vi "Extra_Motor.vi"(7 "refnum name":string="My Motor RefNum", 8 "Back Speed":dbl, 9 "For Speed":dbl, 10 "Backward":bool, 11 "Forward":bool) -> ()   [LabVIEW 2017]
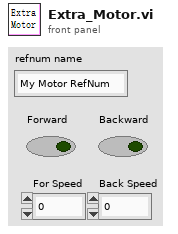
[diagram p1: front panel]
types:
  T1 = typedef "WPI_MotorControlDeviceRef.ctl" = cluster{"DeviceStatus":errorcluster, "Type":T2, "PWM":cluster{"PWM Channel":T3, "DeadBand":T4}, "CAN":cluster{"Device Number":u8, "SetOutput VI Ref":variant, "GetOutput VI Ref":variant, "Enable VI Ref":variant, "Disable VI Ref":variant, "Data":variant}, "Invert":bool, "DIO PWM":cluster{"PWM \"Enable\" Channel":T3, "DIOChannel":T5, "PWM Rate":dbl}}
  T2 = typedef "WPI_MotorControlType.ctl" = enum16{"PWM", "CAN", "DIO PWM"}
  T3 = typedef "FPGA_DIOPWMChannel.ctl" = enum8{"PWM 0", "PWM 1", "PWM 2", "PWM 3", "PWM 4", "PWM 5", "PWM 6", "PWM 7", "PWM 8", "PWM 9", "PWM MXP 0", "PWM MXP 1", "PWM MXP 2", "PWM MXP 3", "PWM MXP 4", "PWM MXP 5", "PWM MXP 6", "PWM MXP 7", "PWM MXP 8", "PWM MXP 9", "Invalid"}
  T4 = typedef "WPI_PWMDeadband.ctl" = cluster{"Name":string, "maxPositivePwm":i32, "minPositivePwm":i32, "centerPwm":i32, "maxNegativePwm":i32, "minNegativePwm":i32, "angularRange":u16}
  T5 = typedef "FPGA_DIOChannel.ctl" = enum8{"DIO 0", "DIO 1", "DIO 2", "DIO 3", "DIO 4", "DIO 5", "DIO 6", "DIO 7", "DIO 8", "DIO 9", "DIO MXP 0", "DIO MXP 1", "DIO MXP 2", "DIO MXP 3", "DIO MXP 4", "DIO MXP 5", "DIO MXP 6", "DIO MXP 7", "DIO MXP 8", "DIO MXP 9", "DIO MXP 10", "DIO MXP 11", "DIO MXP 12", "DIO MXP 13", "DIO MXP 14", "DIO MXP 15", "SPI Port CS1", "SPI Port CS2", "SPI Port CS3", "SPI Port MISO", "SPI Port MOSI", "Invalid"}
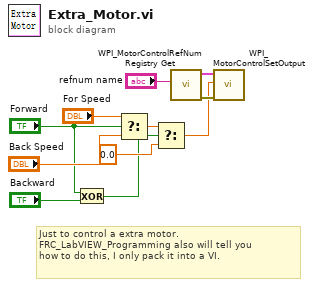
[diagram p0: block diagram]
diagram:
  # "Just to control a extra motor.\nFRC_LabVIEW_Programming also will tell you\nhow to do this, I only pack it into a VI."
  n1 = Exclusive Or(1:"Backward", 2:"Forward") -> (0:w4:bool)
  n2 = Select(t="For Speed", s="Forward", f="Back Speed") -> (s? t:f=w8:dbl)
  n3 = Select(t=w8, s=w4, f=0.0) -> (s? t:f=w1:dbl)
  n4 = call <vilib>:"WPI_MotorControlRefNum Registry Get.vi"("refnum name"="refnum name") -> ("error out"=w3:errorcluster, "MotorControlDevRef"=w2:T1)  [unwired: 9 in]
  n5 = call <vilib>:"WPI_MotorControlSetOutput.vi"("error in (no error)"=w3, "Output"=w1, "MotorControlDevRef"=w2) -> ()  [unwired: 6 in, 3 out]
